vi "Parse Data.vi"(8 "error in":errorcluster, 11 "Data Read":string="0 - \"D03-032 SWV9.02 ESNE03-1120\" H 1721163084.327130 T 25.00 f 7201.79 df 1.42 Fv 15 ph 90 V 0.001 D 1.000 I- 2 I+ 2 Q 0.9824078 fr 8701.3590000 df- 8701.8100000 df+ 8700.8950000 c1 0.190 c2 2.473 Tc 200.00 E 10") -> (0 "error out":errorcluster, 2 "Graph Data out":T1, 3 "Data Out":string[](array[string]))   [LabVIEW 2021]
uses:
  controls/Data for Graph.ctl
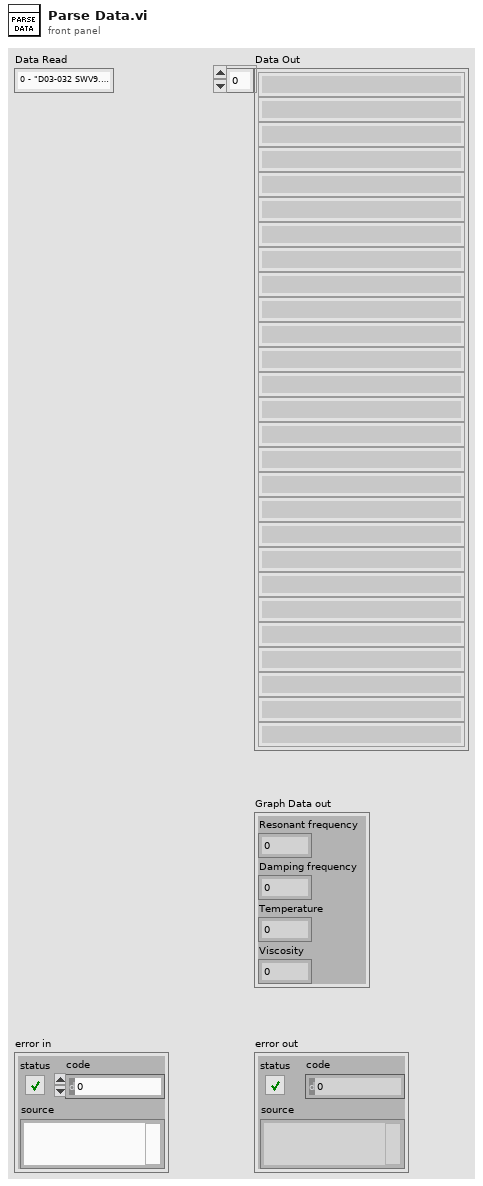
[diagram p1: front panel]
types:
  T1 = typedef "Data for Graph.ctl" = cluster{"Resonant frequency":dbl, "Damping frequency":dbl, "Temperature":dbl, "Viscosity":dbl}
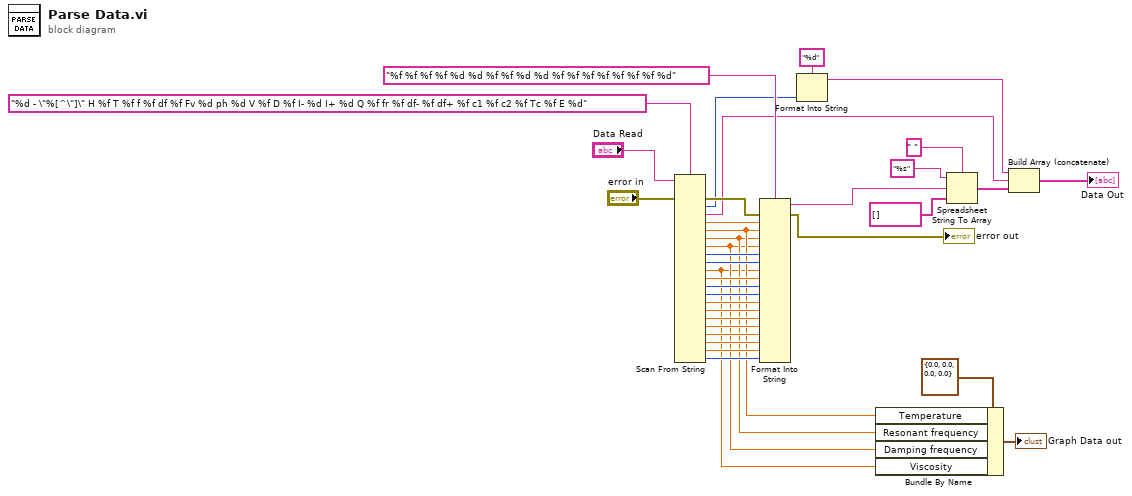
[diagram p0: block diagram]
diagram:
  n1 = Scan From String(format string="%d - \"%[^\"]\" H %f T %f f %f df %f Fv %d ph %d V %f D %f I- %d I+ %d Q %f fr %f df- %f df+ %f c1 %f c2 %f Tc %f E %d", input string="Data Read", error in="error in") -> (error out=w12:errorcluster, output 1=w11:i32, output 2=w7:string, output 3=w32:dbl, output 4=w5:dbl, output 5=w4:dbl, output 6=w3:dbl, output 7=w31:i32, output 8=w30:i32, output 9=w2:dbl, output 10=w29:dbl, output 11=w28:i32, output 12=w27:i32, output 13=w26:dbl, output 14=w25:dbl, output 15=w24:dbl, output 16=w23:dbl, output 17=w22:dbl, output 18=w21:dbl, output 19=w20:dbl, output 20=w19:i32)  [unwired: 21 in, 2 out]
  n2 = Format Into String(format string="%f %f %f %f %d %d %f %f %d %d %f %f %f %f %f %f %f %d", error in=w12, w32, w5, w4, w3, w31, w30, w2, w29, w28, w27, w26, w25, w24, w23, w22, w21, w20, w19) -> (resulting string=w17:string, error out=→"error out":errorcluster)  [unwired: 1 in]
  n3 = Format Into String(format string="%d", w11) -> (resulting string=w8:string)  [unwired: 2 in, 1 out]
  n4 = Bundle By Name(cluster=T1 {"Resonant frequency"=0.0, "Damping frequency"=0.0, "Temperature"=0.0, "Viscosity"=0.0} ("Graph Data"), "Temperature"=w5, "Resonant frequency"=w4, "Damping frequency"=w3, "Viscosity"=w2) -> (→"Graph Data out":T1)
  n5 = Spreadsheet String To Array(delimiter (Tab)=" ", format string="%s", spreadsheet string=w17, array type (2D Dbl)=string[] [] ("format string")) -> (array=w14:string[])
  n6 = Build Array (concatenate)(w8, w7, w14) -> (→"Data Out":string[])
